vi "Elapsed_Time_TMP.vi"() -> ()   [LabVIEW 2017]
uses:
  Robot Global Data.vi
panel:
  out "Time Delta(ms)":u32
  in  "Reset Time":bool
  out "Elapsed Time":u32
  out "Time(sec)":dbl
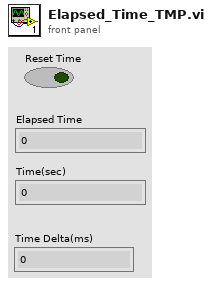
[diagram p1: front panel]
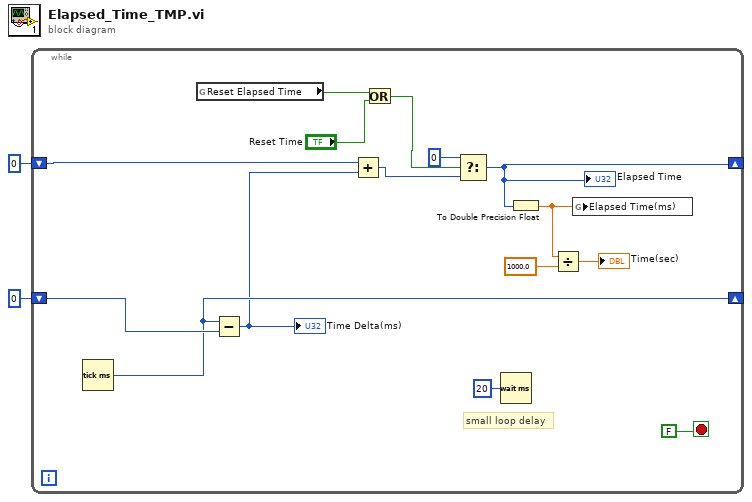
[diagram p0: block diagram]
diagram:
  n1 = while {
    shift-right: [w4] -> _
    shift-left: u32 0 ("millisecond timer value") -> [w15]
    shift-right: [w11] -> _
    shift-left: u32 0 -> [w13]
    stop <- FALSE stop-if-true
    # "small loop delay"
    n2 = Tick Count (ms)() -> (millisecond timer value=w4:u32)
    n3 = global read "Robot Global Data.vi" "Reset Elapsed Time"() -> (w10:bool)
    n4 = Subtract(x=w4, y=w15) -> (x-y=w3:u32)
    "Time Delta(ms)" <- w3
    n5 = Add(x=w13, y=w3) -> (x+y=w14:u32)
    n6 = Or(x=w10, y="Reset Time") -> (x .or. y?=w5:bool)
    n7 = Select(t=u32 0, s=w5, f=w14) -> (s? t:f=w11:u32)
    "Elapsed Time" <- w11
    n8 = Wait (ms)(milliseconds to wait=u32 20) -> ()  [unwired: 1 out]
    n9 = To Double Precision Float(number=w11) -> (double precision float=w8:dbl)
    n10 = Divide(x=w8, y=1000.0) -> (x/y=→"Time(sec)":dbl)
    n11 = global write "Robot Global Data.vi" "Elapsed Time(ms)"(w8) -> ()
  }
